vi "保存报表.vi"(9 "数组":string[][](array[string]), 10 "条码":string, 11 "当前VI路径":path) -> ()   [LabVIEW 2014]
panel:
  out "添加的路径":path
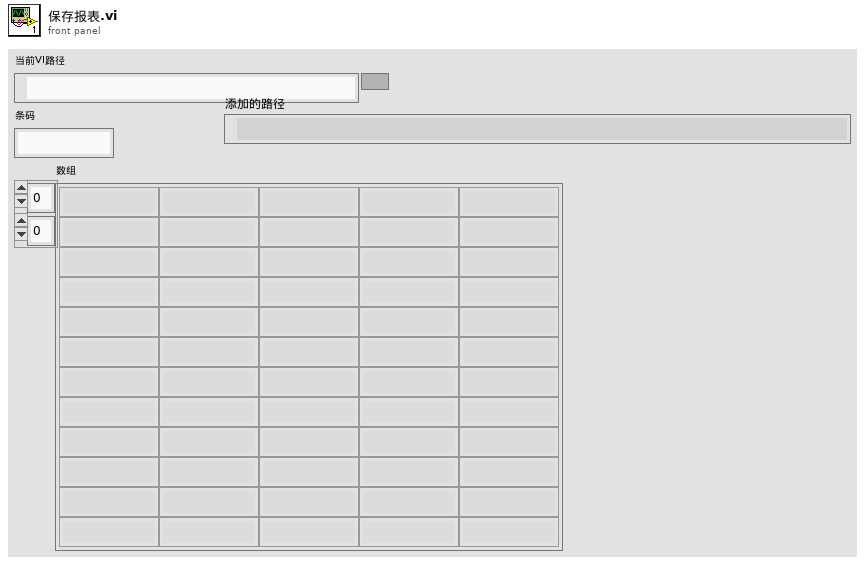
[diagram p1: front panel]
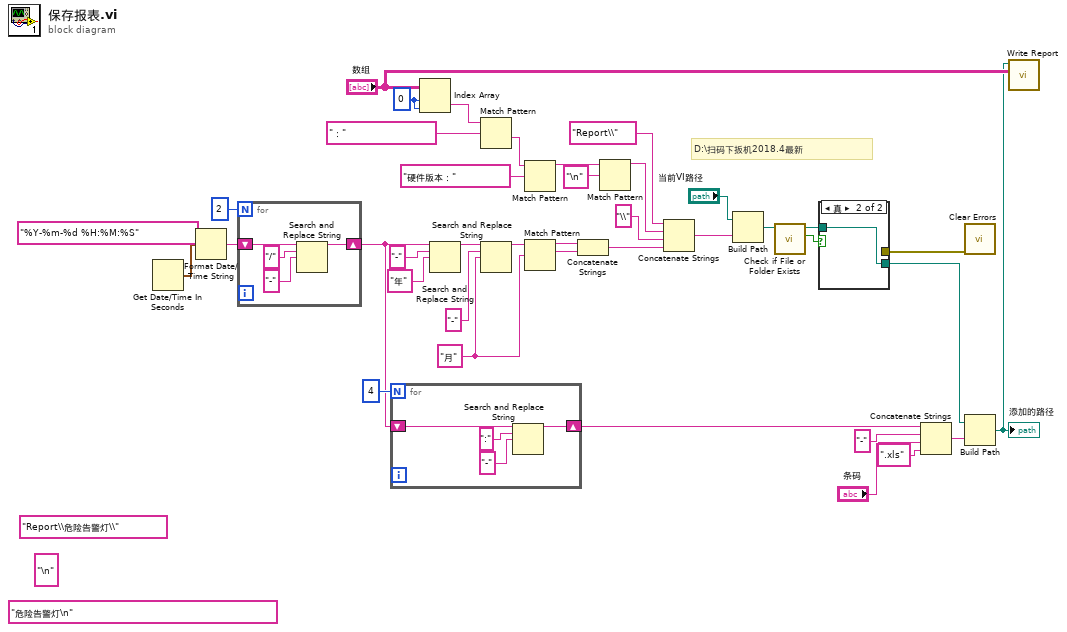
[diagram p0: block diagram]
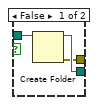
[diagram p2: hidden frame]
diagram:
  (unwired) "Report\\危险告警灯\\" ("连接的字符串")
  (unwired) "\n" ("匹配子字符串")
  (unwired) "危险告警灯\n" ("子字符串之前")
  w24 = "月" ("替换字符串(\"\")")
  w36 = 0 ("索引 (行)")
  # "D:\\扫码下扳机2018.4最新"
  n1 = Get Date/Time In Seconds() -> (seconds since 1Jan1904=w38:timestamp)
  n2 = Format Date/Time String(time format string (%c)="%Y-%m-%d %H:%M:%S" ("时间格式字符串(%c)"), seconds (now)=w38) -> (date/time string=w4:string)  [unwired: 1 in]
  n3 = for {
    N: 2 -> [_]
    shift-right: [w40] -> w3
    shift-left: w4 -> [w43]
    n4 = Search and Replace String(input string=w43, search string="/" ("搜索字符串"), replace string="-" ("替换字符串(\"\")")) -> (result string=w40:string)  [unwired: 5 in, 3 out]
  }
  n5 = for {
    N: 4 -> [_]
    shift-right: [w44] -> w6
    shift-left: w3 -> [w47]
    n6 = Search and Replace String(input string=w47, search string=":" ("搜索字符串"), replace string="-" ("替换字符串(\"\")")) -> (result string=w44:string)  [unwired: 5 in, 3 out]
  }
  n7 = Index Array(array="数组", index (row)=w36, index (col)=w36) -> (element=w35:string)
  n8 = Search and Replace String(input string=w3, search string="-" ("搜索字符串"), replace string="年" ("替换字符串(\"\")")) -> (result string=w27:string)  [unwired: 5 in, 3 out]
  n9 = Match Pattern(string=w35, regular expression="：") -> (after substring=w33:string)  [unwired: 1 in, 3 out]
  n10 = Search and Replace String(input string=w27, search string="-" ("搜索字符串"), replace string=w24) -> (result string=w25:string)  [unwired: 5 in, 3 out]
  n11 = Match Pattern(string=w33, regular expression="硬件版本：") -> (before substring=w12:string)  [unwired: 1 in, 3 out]
  n12 = Match Pattern(string=w25, regular expression=w24) -> (before substring=w23:string, match substring=w22:string)  [unwired: 1 in, 2 out]
  n13 = Concatenate Strings(w23, w22) -> (w7:string)
  n14 = Match Pattern(string=w12, regular expression="\n" ("正则表达式")) -> (before substring=w11:string)  [unwired: 1 in, 3 out]
  n15 = Concatenate Strings("Report\\" ("字符串"), w11, "\\" ("字符串"), w7) -> (w9:string)
  n16 = Build Path(base path="当前VI路径", name or relative path=w9) -> (appended path=w16:path)
  n17 = call <vilib>:"Check if File or Folder Exists.vi"("path"=w16) -> ("file or folder exists?"=w15:bool, "dup path"=w14:path)  [unwired: 8 in, 1 out]
  n18 = case shown="真" w15 {
    tunnel: [w50 w51] -> w13
    tunnel: [w49 _] -> w17
    tunnel: w14 -> [w48 w51]
    frame False {
      n19 = Create Folder(path (use dialog)=w48) -> (created path=w50:path, error out=w49:errorcluster)  [unwired: 2 in, 1 out]
    }
    frame True {
    }
  }
  n20 = Concatenate Strings(w6, "-" ("字符串"), "条码", ".xls" ("字符串")) -> (w18:string)
  n21 = call <vilib>:"Clear Errors.vi"("error in (no error)"=w17) -> ()  [unwired: 5 in, 2 out]
  n22 = Build Path(base path=w13, name or relative path=w18) -> (appended path=w8:path)
  "添加的路径" <- w8
  n23 = call "Write Report.vi"("Data"="数组", "file path"=w8) -> ()  [unwired: 10 in]
